vi "2layer_Neuron.vi"(1 "Offset":dbl, 2 "Weights_2layer":dbl[](array[numeric]), 3 "Array_Out_hx":dbl[](array[numeric])) -> (0 "Output":dbl)   [LabVIEW 2016]
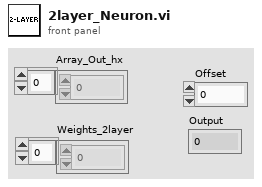
[diagram p1: front panel]
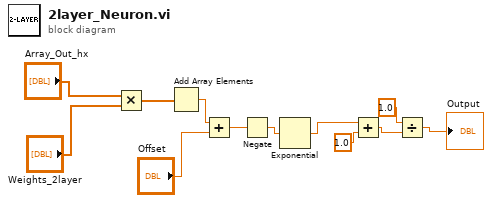
[diagram p0: block diagram]
diagram:
  n1 = Multiply(x="Array_Out_hx", y="Weights_2layer") -> (x*y=w4:dbl[])
  n2 = Add Array Elements(numeric array=w4) -> (sum=w3:dbl)
  n3 = Add(x=w3, y="Offset") -> (x+y=w1:dbl)
  n4 = Negate(x=w1) -> (-x=w9:dbl)
  n5 = Exponential(1:w9) -> (0:w8:dbl)
  n6 = Add(x=w8, y=1.0) -> (x+y=w11:dbl)
  n7 = Divide(x=1.0, y=w11) -> (x/y=→"Output":dbl)
